vi "Event Log - Finished.vi"() -> ()   [LabVIEW 2011]
uses:
  Event Log - Priority.ctl
panel:
  out "VI Started":string
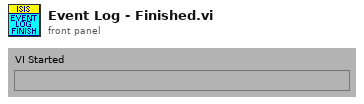
[diagram p1: front panel]
types:
  T1 = typedef "Event Log - Priority.ctl" = enum16{"None", "Log", "SECI and Log"}
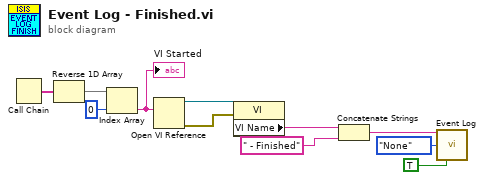
[diagram p0: block diagram]
diagram:
  n1 = Call Chain() -> (call chain=w10:string[])
  n2 = Reverse 1D Array(array=w10) -> (reversed array=w9:string[])
  n3 = Index Array(array=w9, index=0) -> (element=w2:string)
  "VI Started" <- w2
  n4 = Open VI Reference(vi path=w2) -> (vi reference=w7:refnum<vi>, error out=w6:errorcluster)  [unwired: 5 in]
  n5 = property class="VI"(reference=w7, error in=w6) -> ("VI Name"=w5:string)  [unwired: 2 out]
  n6 = Concatenate Strings(w5, " - Finished") -> (w3:string)
  n7 = call "Event Log.vi"("Event log message"=w3, "Priority"=Event_Log_-_Priority."None", "Disconnecting"=TRUE) -> ()  [unwired: 12 in, 1 out]
